vi "Try_Updating_Files.vi"() -> ()   [LabVIEW 2010]
uses:
  Globals/Constants_global.vi
panel:
  out "Files to update":string[][](array[string])
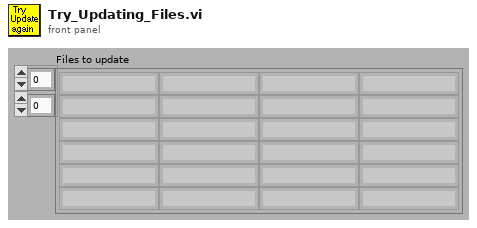
[diagram p1: front panel]
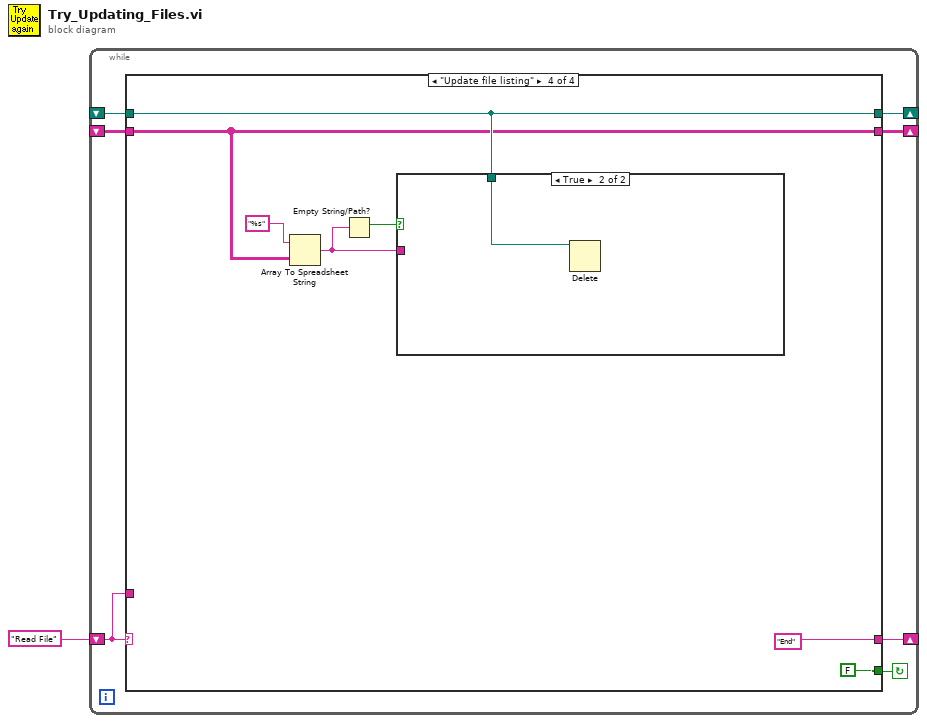
[diagram p0: block diagram]
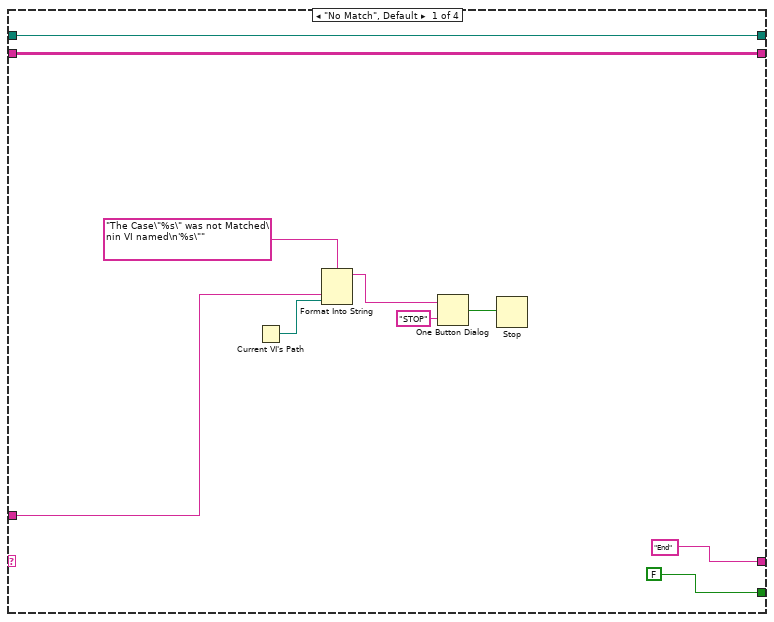
[diagram p2: hidden frame]
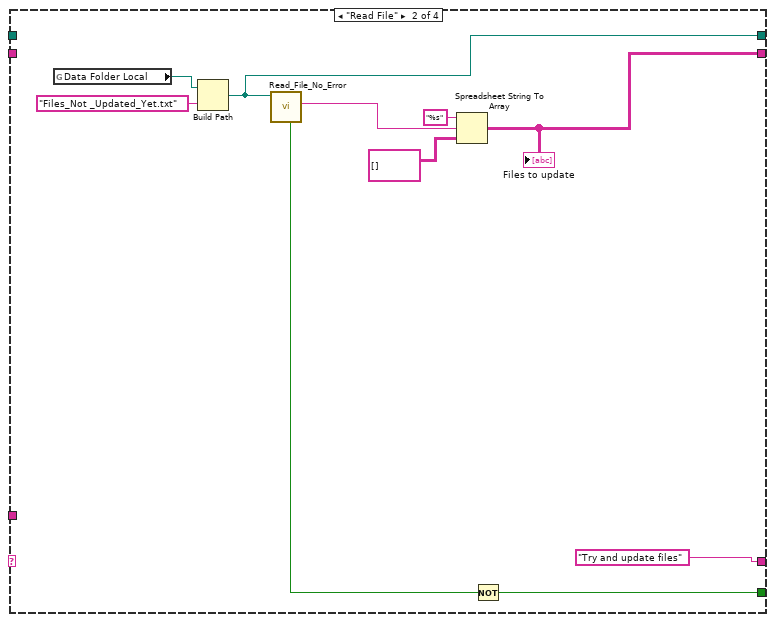
[diagram p3: hidden frame]
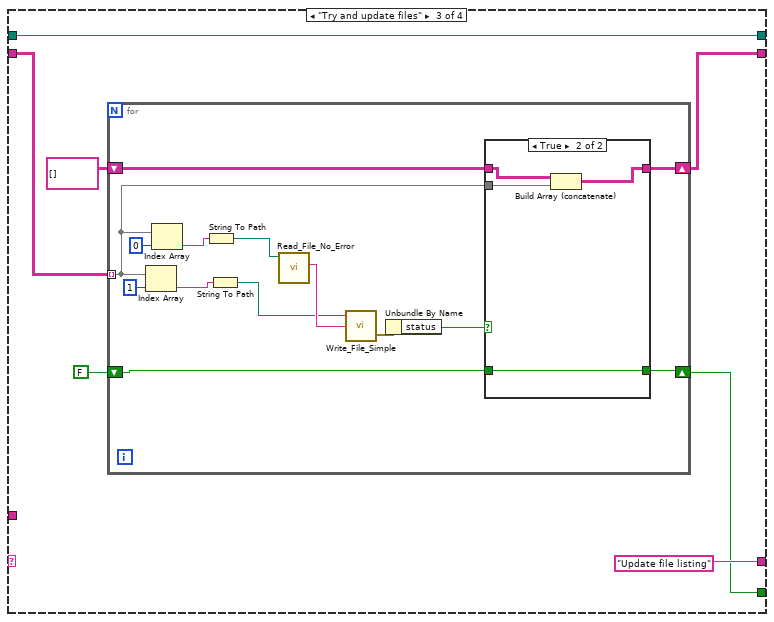
[diagram p4: hidden frame]
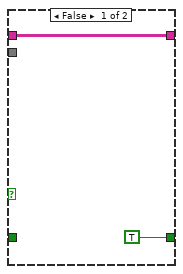
[diagram p5: hidden frame]
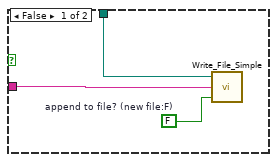
[diagram p6: hidden frame]
diagram:
  n1 = while {
    shift-left: "Read File" -> [w6]
    shift-right: [w7] -> _
    shift-right: [w5] -> _
    shift-left: _ -> [w3]
    shift-right: [w4] -> _
    shift-left: _ -> [w2]
    stop <- w8 continue-if-true
    n2 = case shown="\"Update file listing\"" w6 {
      tunnel: [FALSE w24 w30 FALSE ("status")] -> w8
      tunnel: ["End" "Try and update files" "Update file listing" "End"] -> w7
      tunnel: w6 -> [w13 _ _ _]
      tunnel: [w10 w26 w34 w61] -> w5
      tunnel: [w9 w21 w32 w59] -> w4
      tunnel: w3 -> [w10 _ w34 w61]
      tunnel: w2 -> [w9 _ w31 w59]
      frame "No Match", Default {
        n3 = Current VI's Path() -> (path=w12:path)
        n4 = Format Into String(format string="The Case\"%s\" was not Matched\nin VI named\n'%s\"" ("Format String"), w13, w12) -> (resulting string=w16:string)  [unwired: 2 in, 1 out]
        n5 = One Button Dialog(message=w16, button name ("OK")="STOP") -> (true=w14:bool)
        n6 = Stop(stop? (T)=w14) -> ()
      }
      frame "Read File" {
        n7 = global read "Constants_global.vi" "Data Folder Local"() -> (w28:path)
        n8 = Build Path(base path=w28, name or relative path="Files_Not _Updated_Yet.txt") -> (appended path=w26:path)
        n9 = call "Read_File_No_Error.vi"("Filename"=w26) -> ("Error?"=w25:bool, "string"=w23:string)  [unwired: 2 in, 6 out]
        n10 = Spreadsheet String To Array(format string="%s", spreadsheet string=w23, array type (2D Dbl)=string[][] []) -> (array=w21:string[][])  [unwired: 1 out]
        "Files to update" <- w21
        n11 = Not(x=w25) -> (.not. x?=w24:bool)
      }
      frame "Try and update files" {
        n12 = for {
          tunnel: w31 -> [w40] mode=indexing
          shift-right: [w38] -> w32
          shift-left: string[][] [] -> [w39]
          shift-right: [w37] -> w30
          shift-left: FALSE -> [w36]
          n13 = Index Array(array=w40, index=1) -> (element=w45:string)
          n14 = Index Array(array=w40, index=0) -> (element=w46:string)
          n15 = String To Path(string=w46) -> (path=w44:path)
          n16 = String To Path(string=w45) -> (path=w43:path)
          n17 = call "Read_File_No_Error.vi"("Filename"=w44) -> ("string"=w49:string)  [unwired: 2 in, 7 out]
          n18 = call "Write_File_Simple.vi"("character string"=w49, "file path"=w43) -> ("error out"=w42:errorcluster)  [unwired: 1 in, 1 out]
          n19 = Unbundle By Name(w42) -> ("status"=w41:bool)
          n20 = case shown="True" w41 {
            tunnel: w40 -> [_ w55]
            tunnel: w39 -> [w51 w54]
            tunnel: [w51 w53] -> w38
            tunnel: [TRUE w52] -> w37
            tunnel: w36 -> [_ w52]
            frame False {
            }
            frame True {
              n21 = Build Array (concatenate)(w54, w55) -> (w53:string[][])
            }
          }
        }
      }
      frame "Update file listing" {
        n22 = Array To Spreadsheet String(array=w59, 3:"%s" ("format string")) -> (spreadsheet string=w57:string)  [unwired: 1 out]
        n23 = Empty String/Path?(string/path=w57) -> (empty?=w56:bool)
        n24 = case shown="True" w56 {
          tunnel: w61 -> [w65 w66]
          tunnel: w57 -> [w63 _]
          frame False {
            w64 = FALSE  # append to file? (new file:F)
            n25 = call "Write_File_Simple.vi"("append to file? (new file:F)"=w64, "character string"=w63, "file path"=w65) -> ()  [unwired: 2 out]
          }
          frame True {
            n26 = Delete(path (use dialog)=w66) -> ()  [unwired: 1 in, 6 out]
          }
        }
      }
    }
  }
